vi "Forward Menu Selection.vi"(8 "error in (no error)":errorcluster, 10 "MenuTag":string, 11 "HIJ 4 Alignment Cams App in":refnum<class "HIJ 4 Alignment Cams App.lvclass">) -> (0 "error out":errorcluster, 3 "HIJ 4 Alignment Cams App out":refnum<class "HIJ 4 Alignment Cams App.lvclass">)   [LabVIEW 2014, in "HIJ 4 Alignment Cams App.lvlib" / "HIJ 4 Alignment Cams App.lvclass"]
uses:
  HIJ 4 Alignment Cams App.lvclass
  HIJ 4 Alignment Cams App.lvclass/HIJ 4 Alignment Cams App.ctl
  Applications/HIJ Vision Camera App/HIJ Vision Camera App Messages/Menu Selection Msg/Menu Selection Msg.lvclass/Menu Selection Msg.ctl
  <vilib>/ActorFramework/Message Enqueuer/Message Enqueuer.lvclass/Message Enqueuer.ctl
  <vilib>/ActorFramework/Message Enqueuer/Enqueue.vi
  <vilib>/ActorFramework/Message Priority Queue/Priority Enqueue.vi
  Applications/HIJ Vision Camera App/HIJ Vision Camera App Messages/Menu Selection Msg/Menu Selection Msg.lvclass
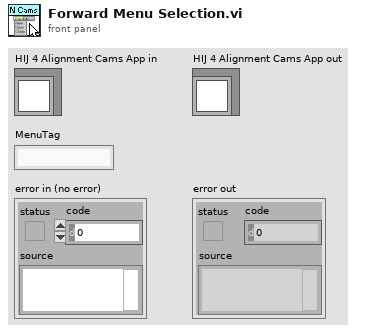
[diagram p1: front panel]
types:
  T1 = typedef "HIJ 4 Alignment Cams App.lvlib/HIJ 4 Alignment Cams App.lvclass/CamAppInfo.ctl" = cluster{"Camera":T2, "App enq":refnum<class "Message Enqueuer.lvclass">, "SubPnl Refnum":refnum<vi>}
  T2 = typedef "IMAQdx.ctl" = refnum<k21>
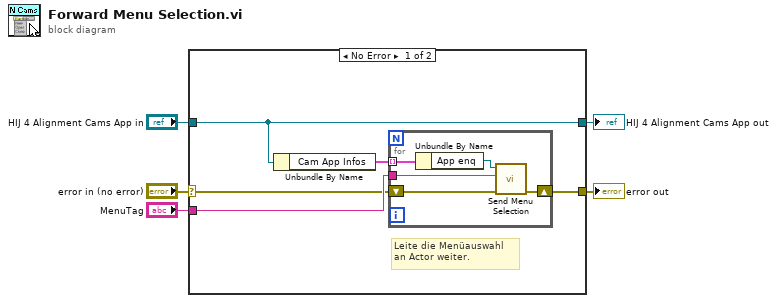
[diagram p0: block diagram]
diagram:
  n1 = case shown="No Error" "error in (no error)" {
    selector: "error in (no error)" -> [w7 w17]
    tunnel: [w6 w17] -> w4
    tunnel: [w10 w16] -> w2
    tunnel: "HIJ 4 Alignment Cams App in" -> [w10 w16]
    tunnel: "MenuTag" -> [w8 _]
    frame No Error {
      # "Leite die Menüauswahl \nan Actor weiter."
      n2 = Unbundle By Name(w10) -> ("Cam App Infos"=w9:T1[])
      n3 = for {
        tunnel: w9 -> [w15] mode=indexing
        tunnel: w8 -> [w13]
        shift-right: [w12] -> w6
        shift-left: w7 -> [w11]
        n4 = Unbundle By Name(w15) -> ("App enq"=w14:refnum<class "Message Enqueuer.lvclass">)
        n5 = call "Send Menu Selection.vi"("error in (no error)"=w11, "MenuTag"=w13, "Message Enqueuer"=w14) -> ("error out"=w12:errorcluster)  [unwired: 7 in, 1 out]
      }
    }
    frame Error {
    }
  }
  "error out" <- w4
  "HIJ 4 Alignment Cams App out" <- w2
